vi "SmoothImage3D.vi"(0 "sector array in":cdb[][][](array[numeric]) format="%.2f", 1 "Override min fill?":bool, 2 "Av size":i32=3, 3 "Min value":dbl format="%.2f") -> (4 "Smoothed Median":dbl[][](array[numeric]) format="%.2f", 5 "Smoothed Sector w/Ave":cdb[][](array[numeric]) format="%.2f", 6 "Var Array":dbl[][](array[numeric]), 7 "Soothed Sector w/ Max neighbor":dbl[][](array[numeric]) format="%.2f")   [LabVIEW 2022 SP3]
uses:
  <vilib>/Analysis/NI_AALBase.lvlib
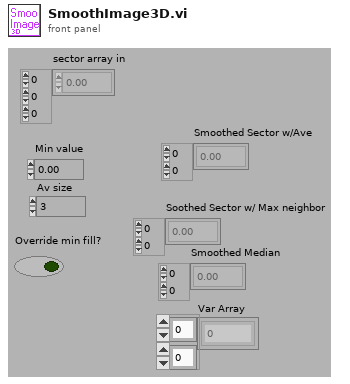
[diagram p1: front panel]
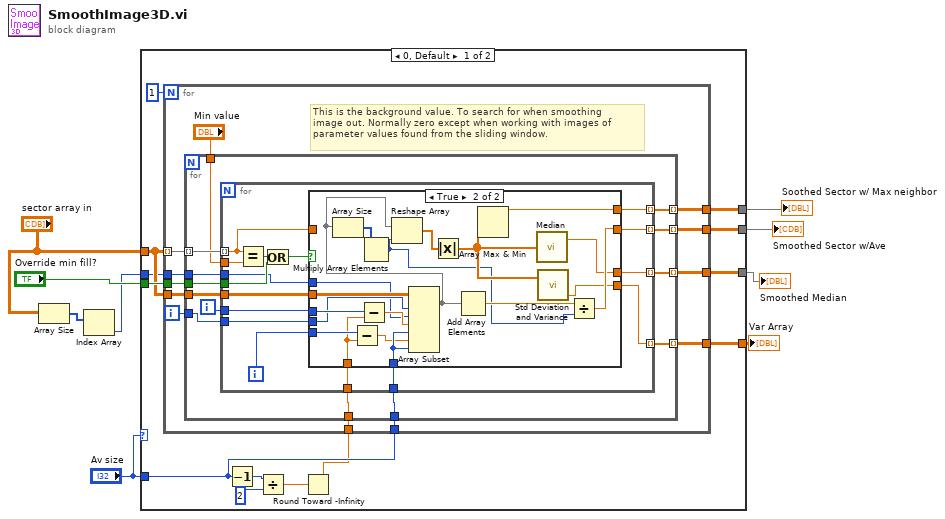
[diagram p0: block diagram]
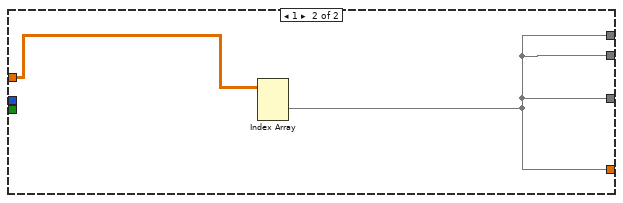
[diagram p3: hidden frame]
diagram:
  n1 = Array Size(array="sector array in") -> (size(s)=w2:i32[])
  n2 = Index Array(array=w2) -> (element=w1:i32)  [unwired: 1 in]
  n3 = case shown="0, Default" "Av size" {
    tunnel: "sector array in" -> [w13 w85]
    tunnel: [w22 w84] -> w9
    tunnel: [w11 w84] -> w8
    tunnel: "Av size" -> [w20 _]
    tunnel: "Override min fill?" -> [w17 _]
    tunnel: [w15 w84] -> w6
    tunnel: [w14 w84] -> w5
    tunnel: w1 -> [w10 _]
    frame 0, Default {
      n4 = Decrement(x=w20) -> (x-1=w16:i32)
      n5 = Divide(x=w16, y=2) -> (x/y=w19:dbl)
      n6 = Round Toward -Infinity(1:w19) -> (0:w18:dbl)
      n7 = for {
        N: 1 -> [_]
        tunnel: w13 -> [w26] mode=indexing
        tunnel: [w34] -> w22
        tunnel: [w33] -> w11
        tunnel: w20 -> [w31]
        tunnel: w18 -> [w30]
        tunnel: w17 -> [w29]
        tunnel: [w28] -> w15
        tunnel: [w27] -> w14
        tunnel: w13 -> [w25]
        tunnel: w10 -> [w23]
        i -> [w24]
        # "This is the background value. To search for when smoothing\nimage out. Normally zero except when working with images of \nparameter values found from the sliding window."
        n8 = for {
          tunnel: w26 -> [w47] mode=indexing
          tunnel: [w46] -> w34 mode=indexing
          tunnel: w25 -> [w45]
          tunnel: [w43] -> w33 mode=indexing
          tunnel: "Min value" -> [w42]
          tunnel: w31 -> [w41]
          tunnel: w30 -> [w40]
          tunnel: w29 -> [w39]
          tunnel: [w38] -> w28 mode=indexing
          tunnel: [w37] -> w27 mode=indexing
          tunnel: w24 -> [w36]
          tunnel: w23 -> [w35]
          i -> [w44]
          n9 = for {
            tunnel: w47 -> [w63] mode=indexing
            tunnel: [w62] -> w46 mode=indexing
            tunnel: w45 -> [w61]
            tunnel: w44 -> [w60]
            tunnel: [w58] -> w43 mode=indexing
            tunnel: w42 -> [w57]
            tunnel: w41 -> [w56]
            tunnel: w40 -> [w55]
            tunnel: w39 -> [w52]
            tunnel: [w51] -> w38 mode=indexing
            tunnel: [w50] -> w37 mode=indexing
            tunnel: w36 -> [w49]
            tunnel: w35 -> [w48]
            i -> [w59]
            n10 = Equal?(x=w63, y=w57) -> (x = y?=w54:bool)
            n11 = Or(x=w54, y=w52) -> (x .or. y?=w53:bool)
            n12 = case shown="True" w53 {
              tunnel: [w64 w77] -> w62
              tunnel: w63 -> [w64 _]
              tunnel: w61 -> [_ w83]
              tunnel: w60 -> [_ w80]
              tunnel: w59 -> [_ w79]
              tunnel: [w64 w81] -> w58
              tunnel: w56 -> [_ w71]
              tunnel: w55 -> [_ w78]
              tunnel: [w64 w76] -> w51
              tunnel: [_ w75] -> w50
              tunnel: w49 -> [_ w68]
              tunnel: w48 -> [_ w65]
              frame False {
              }
              frame True {
                n13 = Subtract(x=w79, y=w78) -> (x-y=w70:dbl)
                n14 = Subtract(x=w80, y=w78) -> (x-y=w69:dbl)
                n15 = Array Subset(array=w83, index (dim 0)=w68, length (dim 0)=w65, index (dim 1)=w69, length (dim 1)=w71, index (dim 2)=w70, length (dim 2)=w71) -> (w73:cdb[][][])
                n16 = Array Size(array=w73) -> (size(s)=w74:i32[])
                n17 = Multiply Array Elements(1:w74) -> (0:w66:i32)
                n18 = Reshape Array(w73, w66) -> (w72:cdb[])
                n19 = Absolute Value(x=w72) -> (abs(x)=w67:dbl[])
                n20 = Add Array Elements(numeric array=w73) -> (sum=w82:cdb)
                n21 = Array Max & Min(array=w67) -> (max value=w81:dbl)  [unwired: 3 out]
                n22 = call <vilib>:"Median.vi"("X"=w67) -> ("median"=w76:dbl)  [unwired: 1 out]
                n23 = call <vilib>:"Std Deviation and Variance.vi"("X"=w67) -> ("variance"=w75:dbl)  [unwired: 1 in, 2 out]
                n24 = Divide(x=w82, y=w66) -> (x/y=w77:cdb)
              }
            }
          }
        }
      }
    }
    frame 1 {
      n25 = Index Array(array=w85) -> (element=w84:cdb[][])  [unwired: 3 in]
    }
  }
  "Smoothed Sector w/Ave" <- w9
  "Soothed Sector w/ Max neighbor" <- w8
  "Smoothed Median" <- w6
  "Var Array" <- w5
